vi "Convert Pane to Screen Coordinates.vi"(6 "error in":errorcluster, 7 "Vertical":i32=20, 8 "Horizontal":i32, 9 "VI ref":refnum<vi>) -> (0 "error out":errorcluster, 1 "Vertical out":i16, 2 "Horizontal out":i16, 3 "VI ref dup":refnum<vi>)   [LabVIEW 2010]
doc: "This function converts Pane Coordinates (used by control property nodes) to Screen Coordinates (used by VI property nodes)."
uses:
  <vilib>/Utility/miscctls.llb/LVPointTypeDef.ctl
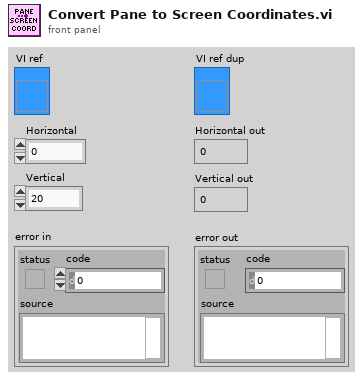
[diagram p1: front panel]
types:
  T1 = typedef "LVPointTypeDef.ctl" = cluster{"Horizontal":i16, "Vertical":i16}
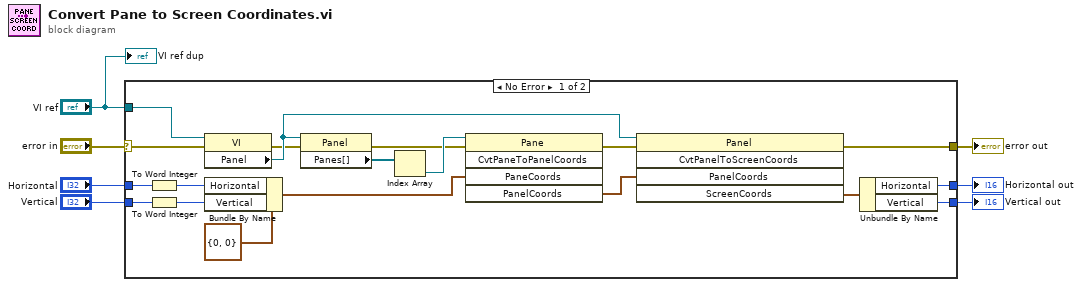
[diagram p0: block diagram]
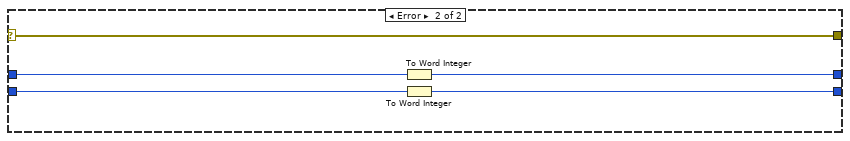
[diagram p2: hidden frame]
diagram:
  n1 = case shown="No Error" "error in" {
    selector: "error in" -> [w21 w31]
    tunnel: [w14 w31] -> w7
    tunnel: "VI ref" -> [w26 _]
    tunnel: "Horizontal" -> [w13 w30]
    tunnel: "Vertical" -> [w12 w29]
    tunnel: [w11 w28] -> w4
    tunnel: [w10 w27] -> w1
    frame No Error {
      n2 = To Word Integer(number=w13) -> (16bit integer=w9:i16)
      n3 = To Word Integer(number=w12) -> (16bit integer=w8:i16)
      n4 = property class="VI"(reference=w26, error in=w21) -> (error out=w18:errorcluster, "Panel"=w19:refnum<vi>)  [unwired: 1 out]
      n5 = Bundle By Name(cluster=T1 {"Horizontal"=0, "Vertical"=0} ("Pane Coordinates"), "Horizontal"=w9, "Vertical"=w8) -> (w15:T1)
      n6 = property class="Panel"(reference=w19, error in=w18) -> (error out=w17:errorcluster, "Panes[]"=w24:refnum<vi>[])  [unwired: 1 out]
      n7 = Index Array(array=w24) -> (element=w23:refnum<vi>)  [unwired: 1 in]
      n8 = invoke class="Pane" method="CvtPaneToPanelCoords"(reference=w23, error in=w17, "PaneCoords"=w15) -> (error out=w20:errorcluster, "PanelCoords"=w22:T1)  [unwired: 2 in, 3 out]
      n9 = invoke class="Panel" method="CvtPanelToScreenCoords"(reference=w19, error in=w20, "PanelCoords"=w22) -> (error out=w14:errorcluster, "ScreenCoords"=w25:T1)  [unwired: 2 in, 3 out]
      n10 = Unbundle By Name(w25) -> ("Horizontal"=w11:i16, "Vertical"=w10:i16)
    }
    frame Error {
      n11 = To Word Integer(number=w30) -> (16bit integer=w28:i16)
      n12 = To Word Integer(number=w29) -> (16bit integer=w27:i16)
    }
  }
  "error out" <- w7
  "Horizontal out" <- w4
  "Vertical out" <- w1
  "VI ref dup" <- "VI ref"
